vi "Create DSF Configuration Session.vi"(8 "error in (no error)":errorcluster, 10 "config data":T1) -> (0 "error out":errorcluster, 3 "DSF Configuration Session out":T15)   [LabVIEW 2017, in "DSF Configuration API.lvlib"]
uses:
  DSF Configuration API.lvlib
  Controls/Session/DSF Configuration Reference.ctl
  Controls/DSF File Format/Internal.DSF Configuration.ctl
  Public/Controls/DSF Version Info.ctl
  Controls/DSF File Format/Internal.DSF Plugin with ID.ctl
  Controls/DSF File Format/Internal.DSF Plugin Info.ctl
  Public/Controls/DSF Timing Info.ctl
  Controls/DSF File Format/Internal.DSF Group with ID.ctl
  Controls/DSF File Format/Internal.DSF Group Info.ctl
  Controls/DSF File Format/Internal.DSF Transfer with ID.ctl
  Controls/DSF File Format/Internal.DSF Transfer Info.ctl
  Controls/DSF File Format/Internal.DSF Channel with ID.ctl
  Controls/DSF File Format/Internal.DSF Channel Info.ctl
  Controls/DSF File Format/Internal.DSF Settings with ID.ctl
  Controls/DSF File Format/Internal.DSF Settings Info.ctl
  Controls/Session/DSF Config Data.ctl
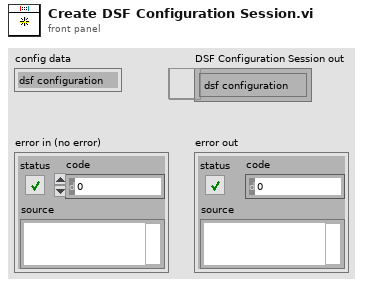
[diagram p1: front panel]
types:
  T1 = typedef "DSF Configuration API.lvlib/DSF Config Data.ctl" = cluster{"dsf configuration":T2, "path":path, "dirty":bool}
  T2 = typedef "DSF Configuration API.lvlib/Internal.DSF Configuration.ctl" = cluster{"dsfversion":T3, "version":T3, "plugins":T4[], "groups":T7[], "transfers":T9[], "channels":T11[], "settings":T13[]}
  T3 = typedef "DSF Configuration API.lvlib/DSF Version Info.ctl" = cluster{"major":u32, "minor":u32, "fix":u32, "build":string}
  T4 = typedef "DSF Configuration API.lvlib/Internal.DSF Plugin with ID.ctl" = cluster{"id":string, "values":T5}
  T5 = typedef "DSF Configuration API.lvlib/Internal.DSF Plugin Info.ctl" = cluster{"type":string, "timing":T6, "group ids":string[], "settings id":string}
  T6 = typedef "DSF Configuration API.lvlib/DSF Timing Info.ctl" = cluster{"priority":i32, "decimation":i32, "offset":i32}
  T7 = typedef "DSF Configuration API.lvlib/Internal.DSF Group with ID.ctl" = cluster{"id":string, "values":T8}
  T8 = typedef "DSF Configuration API.lvlib/Internal.DSF Group Info.ctl" = cluster{"direction":i32, "timing":T6, "transfer ids":string[], "settings id":string}
  T9 = typedef "DSF Configuration API.lvlib/Internal.DSF Transfer with ID.ctl" = cluster{"id":string, "values":T10}
  T10 = typedef "DSF Configuration API.lvlib/Internal.DSF Transfer Info.ctl" = cluster{"byte order":i32, "channel ids":string[], "settings id":string}
  T11 = typedef "DSF Configuration API.lvlib/Internal.DSF Channel with ID.ctl" = cluster{"id":string, "values":T12}
  T12 = typedef "DSF Configuration API.lvlib/Internal.DSF Channel Info.ctl" = cluster{"count":i32, "offset":i32, "data type":i32, "resource path":string, "settings id":string}
  T13 = typedef "DSF Configuration API.lvlib/Internal.DSF Settings with ID.ctl" = cluster{"id":string, "values":T14}
  T14 = typedef "DSF Configuration API.lvlib/Internal.DSF Settings Info.ctl" = cluster{"key":string, "value":string}[]
  T15 = typedef "DSF Configuration API.lvlib/DSF Configuration Reference.ctl" = refnum<data-value>
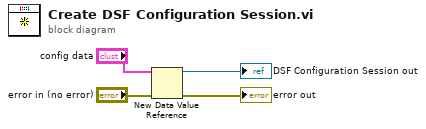
[diagram p0: block diagram]
diagram:
  n1 = New Data Value Reference(data value="config data", error in="error in (no error)") -> (data value reference=→"DSF Configuration Session out":refnum<data-value>, error out=→"error out":errorcluster)
